vi "FGV user laser 1 status.vi"(7 "FGV Actions":enum16{"Get", "Set"}(ring), 8 "error in (no error)":errorcluster, 11 "Laser status IN":T1) -> (0 "error out":errorcluster, 3 "Laser Status OUT":T1)   [LabVIEW 2017]
uses:
  Coherent Control/Type defs/laser status data.ctl
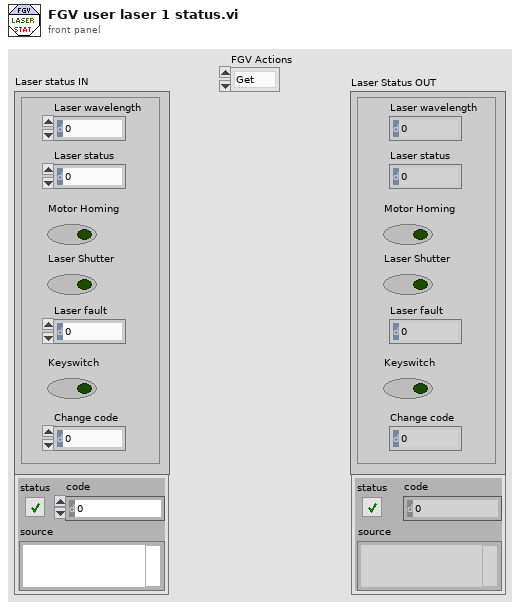
[diagram p1: front panel]
types:
  T1 = typedef "laser status data.ctl" = cluster{"Laser wavelength":i32, "Laser status":u8, "Motor Homing":bool, "Laser Shutter":bool, "Laser fault":u8, "Keyswitch":bool, "Change code":u8}
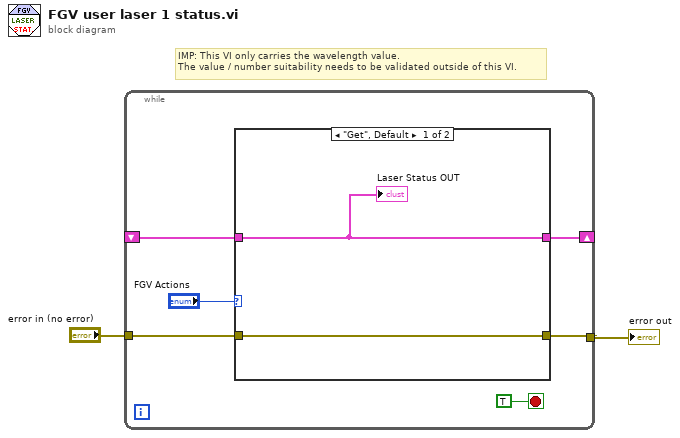
[diagram p0: block diagram]
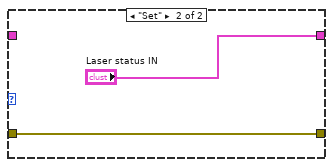
[diagram p2: hidden frame]
diagram:
  # "IMP: This VI only carries the wavelength value.\nThe value / number suitability needs to be validated outside of this VI."
  n1 = while {
    shift-right: [w6] -> _
    shift-left: _ -> [w5]
    tunnel: "error in (no error)" -> [w4]
    tunnel: [w3] -> w1
    stop <- TRUE stop-if-true
    n2 = case shown="\"Get\", Default" "FGV Actions" {
      tunnel: [w10 "Laser status IN"] -> w6
      tunnel: w5 -> [w10 _]
      tunnel: w4 -> [w9 w12]
      tunnel: [w9 w12] -> w3
      frame "Get", Default {
        "Laser Status OUT" <- w10
      }
      frame "Set" {
      }
    }
  }
  "error out" <- w1
